vi "Get Terminal Refs for Unbundle By Name.vi"(8 "error in (no error)":errorcluster, 10 "object refnum":refnum<vi>, 11 "Setter Generator In":refnum<class "Setter Generator.lvclass">) -> (0 "error out":errorcluster, 2 "reference out":refnum<vi>, 3 "Setter Generator Out":refnum<class "Setter Generator.lvclass">)   [LabVIEW 2020, in "Method Generation.lvlib" / "Setter Generator.lvclass"]
uses:
  Setter Generator.lvclass
  Setter Generator.lvclass/Setter Generator.ctl
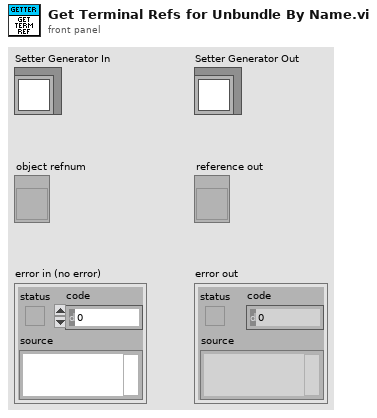
[diagram p1: front panel]
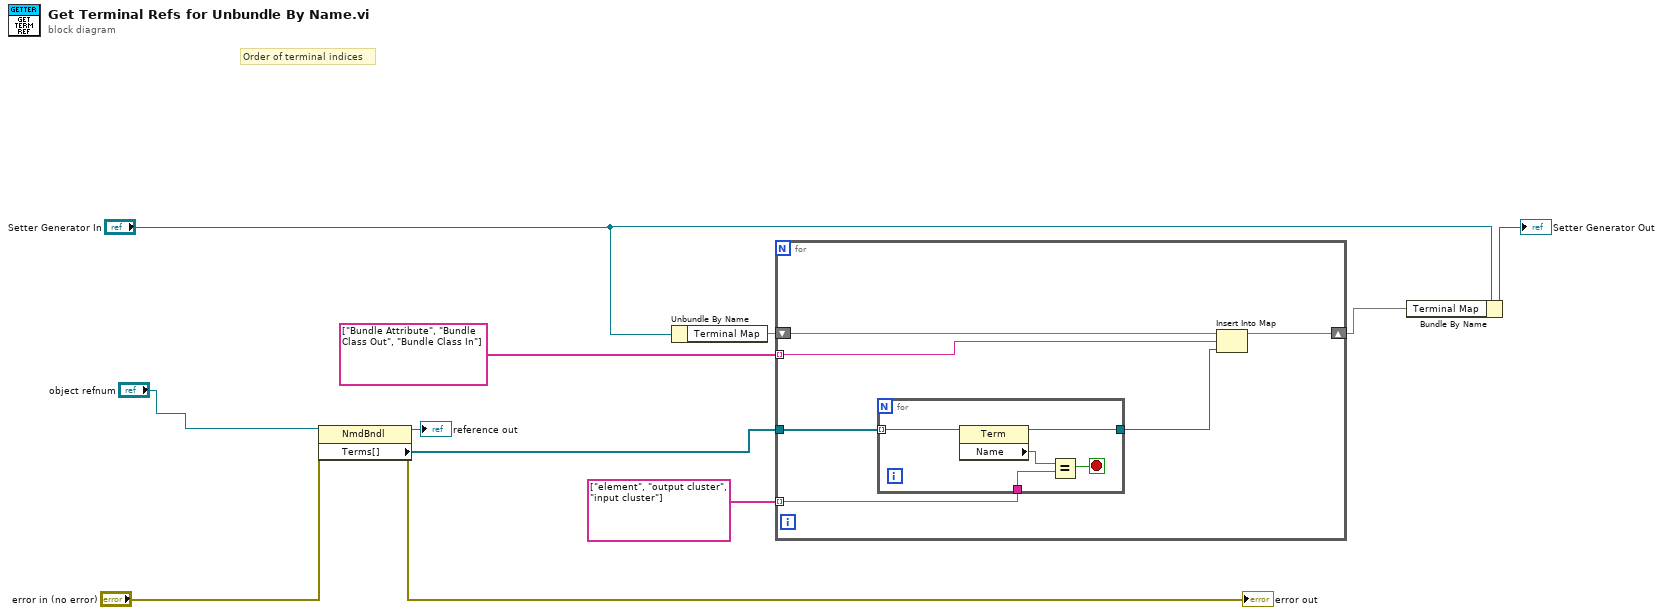
[diagram p0: block diagram]
diagram:
  # "Order of terminal indices"
  n1 = property class="NmdBndl"(reference="object refnum", error in="error in (no error)") -> (reference out=→"reference out":refnum<vi>, error out=→"error out":errorcluster, "Terms[]"=w3:refnum<vi>[])
  n2 = Unbundle By Name("Setter Generator In") -> ("Terminal Map"=w7:map{string, refnum<vi>})
  n3 = for {
    tunnel: w3 -> [w14]
    tunnel: string[] ["Bundle Attribute", "Bundle Class Out", "Bundle Class In"] -> [w16] mode=indexing
    shift-right: [w15] -> w6
    shift-left: w7 -> [w17]
    tunnel: string[] ["element", "output cluster", "input cluster"] -> [w12] mode=indexing
    n4 = for {
      tunnel: w14 -> [w22] mode=indexing
      tunnel: [w21] -> w13
      tunnel: w12 -> [w18]
      stop <- w20 stop-if-true
      n5 = property class="Term"(reference=w22) -> (reference out=w21:refnum<vi>, "Name"=w19:string)  [unwired: 1 in, 1 out]
      n6 = Equal?(x=w19, y=w18) -> (x = y?=w20:bool)
    }
    n7 = Insert Into Map(map in=w17, key=w16, value=w13) -> (map out=w15:map{string, refnum<vi>})  [unwired: 2 out]
  }
  n8 = Bundle By Name(cluster="Setter Generator In", "Terminal Map"=w6) -> (→"Setter Generator Out":refnum<class "Setter Generator.lvclass">)
